vi "Fdx Create Session (Rx-VL-Oriented).vi"(6 "PortMap":u32, 8 "error in (no error)":errorcluster, 9 "DefaultPayloadMode":u32(ring) items=["FDX_PAYLOAD_FULL", "FDX_PAYLOAD_IP_EXT", "FDX_PAYLOAD_IP", "FDX_PAYLOAD_MAC"], 10 "port":u32, 11 "board":u32) -> (0 "error out":errorcluster, 1 "GlbMonBufferSizeOut":u32, 2 "PortInitOut":T1 {"PortConfig" items=["FDX_SINGLE", "FDX_REDUNDANT"]}, 3 "InstrumentHandle_port out":u32, 4 "Duplicated":bool, 5 "InstrumentHandle_board out":u32)   [LabVIEW 2020, in "AIM664LV.lvlib"]
doc: "Creates a session to the port and board and instantiate a VL-Oriented Receive (Rx) to it. Use DefaultPayloadMode to specify how to define the type of data to be received."
uses:
  AIM664LV.lvlib
  _controls/hwEntry_actions.ctl
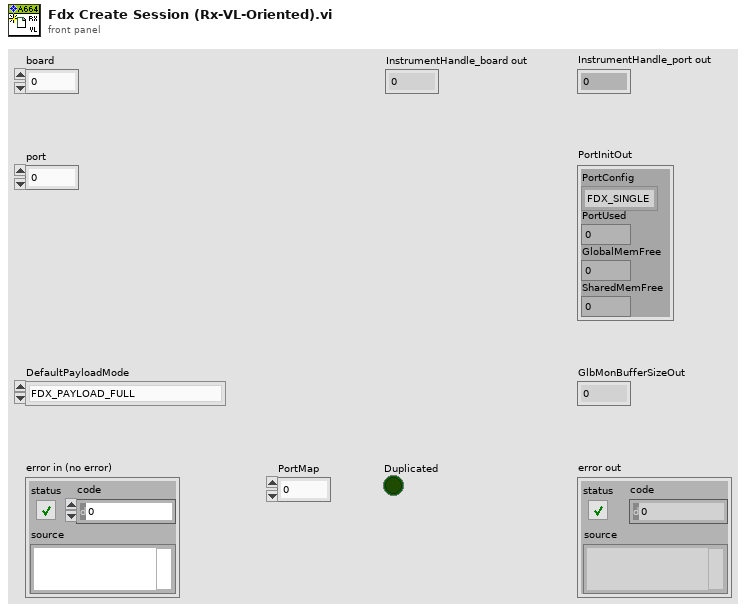
[diagram p1: front panel]
types:
  T1 = cluster{"PortConfig":u32, "PortUsed":u32, "GlobalMemFree":u32, "SharedMemFree":u32}
  T2 = typedef "AIM664LV.lvlib/hwEntry_actions.ctl" = enum16{"Init Port", "Init Board", "Relase Port", "Release Board"}
  T3 = typedef "AIM664LV.lvlib/hwEntry_handleValidityFlag.ctl" = cluster{"boardHandleValid":bool, "portHandleValid":bool}
  T4 = cluster{"ReceiveMode":u32, "DefaultPayloadMode":u32, "DefaultCronoMode":u32, "GlbMonBufferSizeIn":u32, "RerosDefaultOutputPortmap":u32}
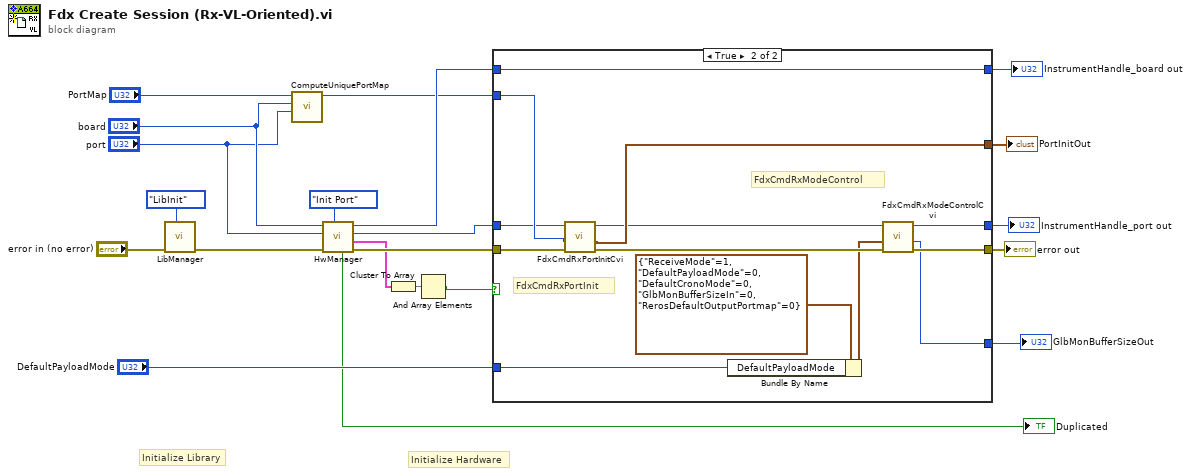
[diagram p0: block diagram]
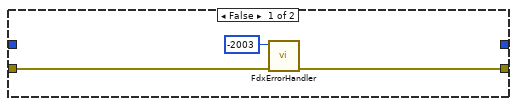
[diagram p2: hidden frame]
diagram:
  # "Initialize Hardware"
  # "Initialize Library"
  n1 = call "LibManager.vi"("action"=enum16{"LibInit", "LibExit"}."LibInit", "error in (no error)"="error in (no error)") -> ("error out"=w19:errorcluster)  [unwired: 7 in, 2 out]
  n2 = call "ComputeUniquePortMap.vi"("port"="port", "board"="board", "PortMap In"="PortMap") -> ("PortMap out"=w8:u32)  [unwired: 8 in]
  n3 = call "HwManager.vi"("action (Init)"=hwEntry_actions."Init Port" ("action"), "error in (no error)"=w19, "port"="port", "board"="board") -> ("error out"=w18:errorcluster, "validityFlag"=w2:T3, "InstrumentHandle_port out"=w11:u32, "InstrumentHandle_board out"=w12:u32, "Duplicated"=→"Duplicated":bool)  [unwired: 3 in]
  n4 = Cluster To Array(cluster=w2) -> (array=w3:bool[])
  n5 = And Array Elements(Boolean array=w3) -> (logical AND=w1:bool)
  n6 = case shown="True" w1 {
    tunnel: w18 -> [w23 w37]
    tunnel: w11 -> [_ w35]
    tunnel: [w22 w31] -> w17
    tunnel: w8 -> [_ w36]
    tunnel: [_ w34] -> w16
    tunnel: w12 -> [_ w25]
    tunnel: [_ w26] -> w15
    tunnel: "DefaultPayloadMode" -> [_ w28]
    tunnel: [_ w27] -> w13
    tunnel: [_ w25] -> w4
    frame False {
      n7 = call "FdxErrorHandler.vi"("error in"=w23, "AIM Error"=-2003) -> ("error out"=w22:errorcluster)  [unwired: 9 in]
    }
    frame True {
      # "FdxCmdRxModeControl"
      # "FdxCmdRxPortInit"
      n8 = call "FdxCmdRxPortInitCvi.vi"("error in"=w37, "PortMap"=w36, "InstrumentHandle_port in"=w35) -> ("error out"=w33:errorcluster, "PortInitOut"=w34:T1, "InstrumentHandle_port out"=w32:u32)  [unwired: 6 in]
      n9 = Bundle By Name(cluster=T4 {"ReceiveMode"=1, "DefaultPayloadMode"=0, "DefaultCronoMode"=0, "GlbMonBufferSizeIn"=0, "RerosDefaultOutputPortmap"=0} ("RxModeControlIn"), "DefaultPayloadMode"=w28) -> (w29:T4)
      n10 = call "FdxCmdRxModeControlCvi.vi"("error in"=w33, "RxModeControlIn"=w29, "InstrumentHandle_port in"=w32) -> ("error out"=w31:errorcluster, "GlbMonBufferSizeOut"=w27:u32, "InstrumentHandle_port out"=w26:u32)  [unwired: 6 in]
    }
  }
  "error out" <- w17
  "PortInitOut" <- w16
  "InstrumentHandle_port out" <- w15
  "GlbMonBufferSizeOut" <- w13
  "InstrumentHandle_board out" <- w4
